vi "To String.vi"(7 "Formatting":enum16{"plain", "fancy"}(ring), 8 "error in":errorcluster, 11 "Orient3d in":refnum<class "Orient3d.lvclass">) -> (0 "error out":errorcluster, 2 "Orient3d String":string, 3 "Orient3d out":refnum<class "Orient3d.lvclass">)   [LabVIEW 2024, in "Orient3d.lvclass"]
uses:
  Orient3d.lvclass
  Orient3d.lvclass/Orient3d.ctl
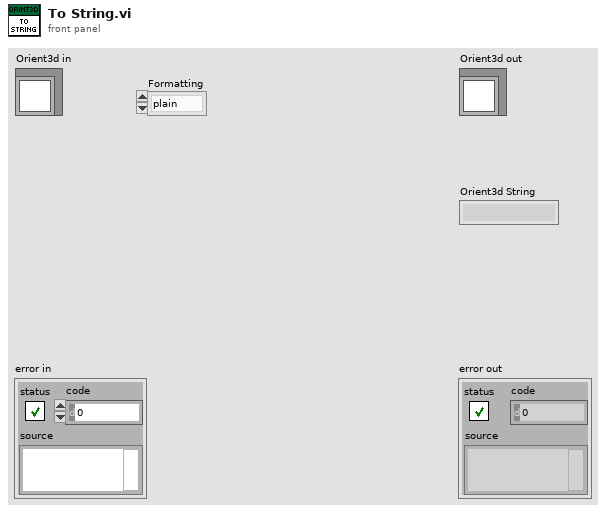
[diagram p1: front panel]
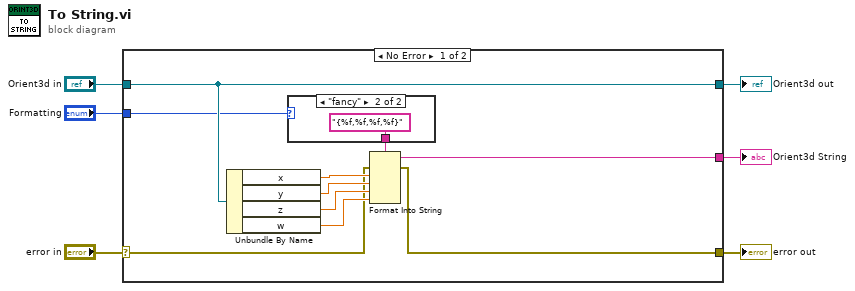
[diagram p0: block diagram]
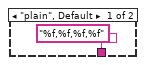
[diagram p2: hidden frame]
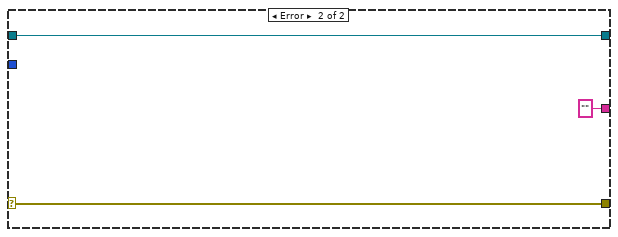
[diagram p3: hidden frame]
diagram:
  n1 = case shown="No Error" "error in" {
    selector: "error in" -> [w10 w21]
    tunnel: [w9 w21] -> w5
    tunnel: [w16 w20] -> w3
    tunnel: "Orient3d in" -> [w16 w20]
    tunnel: [w8 ""] -> w2
    tunnel: "Formatting" -> [w7 _]
    frame No Error {
      n2 = Unbundle By Name(w16) -> ("x"=w14:dbl, "y"=w13:dbl, "z"=w12:dbl, "w"=w11:dbl)
      n3 = case shown="\"fancy\"" w7 {
        tunnel: ["%f,%f,%f,%f" ("format string") "{%f,%f,%f,%f}" ("format string")] -> w15
        frame "plain", Default {
        }
        frame "fancy" {
        }
      }
      n4 = Format Into String(format string=w15, error in=w10, w14, w13, w12, w11) -> (resulting string=w8:string, error out=w9:errorcluster)  [unwired: 1 in]
    }
    frame Error {
    }
  }
  "error out" <- w5
  "Orient3d out" <- w3
  "Orient3d String" <- w2
